vi "LEMP_realtime_v4.vi"() -> ()   [LabVIEW 2019]
uses:
  <vilib>/Analysis/7linalg.llb/Eigenvalue and Vectors Output Option.ctl
  <vilib>/Analysis/baseanly.llb/Matrix Type of Inverse Matrix.ctl
  <vilib>/Analysis/baseanly.llb/Mean (DBL).vi
  <vilib>/Analysis/4window.llb/Hanning Window (DBL).vi
  <vilib>/Analysis/5stat.llb/RMS (DBL).vi
  <vilib>/Analysis/2dsp.llb/Real FFT.vi
  <vilib>/Analysis/7linalg.llb/Real Generalized Eigenvalues and Vectors.vi
  <vilib>/Analysis/7linalg.llb/Real Cholesky Factorization.vi
  <vilib>/Analysis/4window.llb/AllCosWindow (DBL).vi
  <vilib>/Analysis/baseanly.llb/Full Cholesky Factorization.vi
  <vilib>/Analysis/baseanly.llb/Full Real Matrix Cholesky Factorization.vi
  <vilib>/Analysis/Matrix/Numeric/Conversions/Array To Matrix - RA2.vi
  <vilib>/Analysis/baseanly.llb/Real Inverse Matrix.vi
  <vilib>/Analysis/Matrix/Numeric/Multiply/Multiply - RM,RM.vi
  <vilib>/Analysis/7linalg.llb/Real Eigenvalues and Vectors.vi
  <vilib>/Analysis/Matrix/Numeric/Add/Add - RM,RM.vi
  <vilib>/gmath/statdist.llb/Normal Moments.vi
  <vilib>/gmath/NI_Gmath.lvlib
  <vilib>/Analysis/NI_AALPro.lvlib
  <vilib>/Analysis/Matrix/NI_Matrix.lvlib
  <vilib>/Analysis/NI_AALBase.lvlib
panel:
  out "min value":dbl=40.777955555555565
  out "max value":dbl=69.90506666666668
  in  "MASTER":bool
  in  "Tab Control":T1(tab)=enum."Check"
  out "Cycle time (ms)":dbl=0.147275536505731
  out "1st Nat. Freq. (Hz) 2":dbl=40.777955555555565 format="%#_5g"
  out "FEA Frequencies":dbl[](array[numeric])=[47.056894447356875, 51.47067845292848, 50.76081786160022]
  out "Acceleration Data":dbl[](graph) caption="Accelorometer data"
  in  "Real-Time plotting":bool
  out "Probability Density Function":cluster{i32[], dbl[]}(graph)={[9, 10, 11, 12, 13, 14, 15, 16, 17, 18, 19, 20, 21, 22, 23, 24, 25, 26], [0.09171563397251428, 0.12108231855717679, 0.143041857841436, 0.1512135165862316, 0.143041857841436, 0.12108231855717679, 0.09171563397251428, 0.062165735159412254, 0.03770542435775916, 0.020464524096401888, 0.009939041952144324, 0.004319489826678621, 0.0016798304322918924, 0.0005845793791312176, 0.00018203990329545533, 5.072648364839732e-05, 1.2648760741233286e-05, 2.8223200098705454e-06]}
  out "FFT":dbl[](graph)
  out "Frequencies":dynamicdata(graph)=[{"t0"=timestamp(0 s since 1904-01-01), "dt"=1.0, "Y"=array[322 elements]}, {"t0"=timestamp(0 s since 1904-01-01), "dt"=1.0, "Y"=array[322 elements]}]
  out "Position":dynamicdata(graph)=[{"t0"=timestamp(0 s since 1904-01-01), "dt"=1.0, "Y"=[10.0, 12.0, 10.0, 10.0, 10.0, 9.0, 10.0, 12.0, 10.0, 9.0, 9.0, 12.0, 10.0, 16.0, 11.0, 14.0, 14.0, 12.0, 12.0, 12.0, 12.0, 14.0, 14.0, 11.0, 12.0, 12.0, 12.0, 12.0, 12.0, 10.0, 12.0, 14.0, 13.0, 16.0, 14.0, 13.0, 16.0, 14.0, 11.0, 11.0, 16.0, 18.0, 11.0, 10.0, 10.0, 12.0, 10.0, 10.0, 12.0, 12.0, 10.0, 12.0, 10.0, 10.0, 10.0, 10.0, 12.0, 9.0, 11.0, 13.0, 15.0, 15.0, 16.0, 18.0, 15.0, 15.0, 17.0, 15.0, 20.0, 18.0, 15.0, 15.0, 11.0, 11.0, 11.0, 12.0, 9.0, 10.0, 10.0, 10.0, 10.0, 12.0, 14.0, 10.0, 12.0, 12.0, 10.0, 10.0, 10.0, 10.0, 10.0, 10.0, 9.0, 10.0, 12.0, 9.0, 9.0, 14.0, 11.0, 13.0, 15.0, 19.0, 19.0, 17.0, 17.0, 17.0, 21.0, 19.0, 26.0, 26.0, 26.0, 26.0, 24.0, 26.0, 24.0, 24.0, 21.0, 20.0, 20.0, 20.0, 22.0, 14.0, 16.0, 18.0, 18.0, 12.0, 10.0, 12.0, 12.0, 12.0, 16.0, 14.0, 10.0, 14.0, 16.0, 16.0, 20.0, 20.0, 22.0, 22.0, 26.0, 21.0, 19.0, 19.0, 15.0, 19.0, 19.0, 19.0, 19.0, 17.0, 20.0, 24.0, 23.0, 21.0, 21.0, 26.0, 26.0, 26.0, 26.0, 24.0, 24.0, 22.0, 20.0, 22.0, 24.0, 22.0, 24.0, 20.0, 17.0, 18.0, 16.0, 13.0, 14.0, 14.0, 12.0, 10.0, 9.0, 10.0, 11.0, 17.0, 17.0, 24.0, 21.0, 23.0, 24.0, 19.0, 21.0, 25.0, 23.0, 26.0, 25.0, 25.0, 23.0, 23.0, 21.0, 23.0, 25.0, 21.0, 26.0, 24.0, 22.0, 18.0, 14.0, 12.0, 12.0, 12.0, 10.0, 12.0, 10.0, 9.0, 10.0, 10.0, 12.0, 11.0, 10.0, 12.0, 10.0, 10.0, 10.0, 10.0, 10.0, 10.0, 10.0, 9.0, 12.0, 12.0, 11.0, 13.0, 14.0, 12.0, 12.0, 12.0, 10.0, 10.0, 12.0, 10.0, 10.0, 10.0, 9.0, 9.0, 10.0, 12.0, 12.0, 18.0, 14.0, 18.0, 15.0, 12.0, 12.0, 12.0, 14.0, 11.0, 12.0, 12.0, 12.0, 11.0, 10.0, 10.0, 9.0, 10.0, 14.0, 16.0, 12.0, 12.0, 13.0, 13.0, 15.0, 13.0, 14.0, 9.0, 9.0, 10.0, 10.0, 9.0, 10.0, 11.0, 10.0, 10.0, 12.0, 11.0, 14.0, 14.0, 12.0, 12.0, 10.0, 13.0, 15.0, 13.0, 15.0, 15.0, 21.0, 19.0, 16.0, 16.0, 14.0, 16.0, 14.0, 12.0, 10.0, 10.0, 10.0, 10.0, 14.0, 22.0, 24.0, 22.0, 26.0, 22.0, 20.0, 20.0, 19.0, 21.0, 21.0, 17.0, 19.0, 17.0, 16.0, 17.0, 14.0, 12.0, 12.0, 10.0]}, {"t0"=timestamp(0 s since 1904-01-01), "dt"=1.0, "Y"=[9.0, 9.0, 9.0, 10.0, 11.0, 11.0, 12.0, 12.0, 12.0, 12.0, 11.0, 11.0, 10.0, 10.0, 9.0, 9.0, 9.0, 9.0, 10.0, 10.0, 11.0, 11.0, 11.0, 12.0, 12.0, 13.0, 13.0, 14.0, 14.0, 14.0, 14.0, 14.0, 15.0, 15.0, 15.0, 14.0, 13.0, 13.0, 12.0, 11.0, 10.0, 10.0, 10.0, 9.0, 9.0, 9.0, 9.0, 9.0, 10.0, 11.0, 11.0, 12.0, 12.0, 13.0, 14.0, 15.0, 16.0, 16.0, 16.0, 17.0, 17.0, 17.0, 17.0, 17.0, 17.0, 17.0, 16.0, 16.0, 15.0, 15.0, 14.0, 13.0, 12.0, 11.0, 11.0, 10.0, 10.0, 10.0, 9.0, 9.0, 9.0, 9.0, 9.0, 9.0, 9.0, 10.0, 11.0, 12.0, 12.0, 13.0, 14.0, 14.0, 15.0, 15.0, 16.0, 17.0, 18.0, 19.0, 19.0, 19.0, 20.0, 20.0, 20.0, 20.0, 20.0, 19.0, 19.0, 19.0, 18.0, 18.0, 17.0, 16.0, 15.0, 15.0, 14.0, 13.0, 12.0, 11.0, 11.0, 10.0, 10.0, 10.0, 9.0, 9.0, 9.0, 9.0, 9.0, 10.0, 10.0, 11.0, 12.0, 13.0, 14.0, 15.0, 16.0, 18.0, 19.0, 20.0, 21.0, 21.0, 22.0, 22.0, 22.0, 23.0, 23.0, 23.0, 23.0, 23.0, 22.0, 22.0, 22.0, 21.0, 21.0, 20.0, 19.0, 18.0, 16.0, 15.0, 14.0, 13.0, 12.0, 12.0, 12.0, 11.0, 10.0, 10.0, 9.0, 9.0, 9.0, 9.0, 10.0, 10.0, 11.0, 12.0, 13.0, 15.0, 16.0, 18.0, 20.0, 21.0, 22.0, 23.0, 24.0, 25.0, 25.0, 25.0, 25.0, 25.0, 25.0, 25.0, 24.0, 23.0, 22.0, 21.0, 20.0, 19.0, 17.0, 15.0, 14.0, 13.0, 12.0, 11.0, 10.0, 10.0, 9.0, 9.0, 9.0, 9.0, 9.0, 9.0, 9.0, 9.0, 9.0, 9.0, 9.0, 9.0, 9.0, 10.0, 11.0, 11.0, 10.0, 9.0, 9.0, 9.0, 9.0, 9.0, 9.0, 9.0, 9.0, 9.0, 9.0, 9.0, 9.0, 9.0, 9.0, 9.0, 9.0, 9.0, 9.0, 9.0, 10.0, 13.0, 14.0, 13.0, 11.0, 10.0, 9.0, 9.0, 9.0, 9.0, 9.0, 9.0, 9.0, 9.0, 9.0, 9.0, 9.0, 9.0, 9.0, 9.0, 9.0, 10.0, 14.0, 16.0, 17.0, 14.0, 12.0, 10.0, 9.0, 9.0, 9.0, 9.0, 9.0, 9.0, 9.0, 9.0, 9.0, 9.0, 9.0, 9.0, 9.0, 9.0, 10.0, 14.0, 18.0, 19.0, 20.0, 18.0, 14.0, 10.0, 9.0, 9.0, 9.0, 9.0, 9.0, 9.0, 9.0, 9.0, 9.0, 9.0, 9.0, 9.0, 9.0, 9.0, 9.0, 10.0, 13.0, 18.0, 22.0, 22.0, 19.0, 15.0, 12.0, 10.0, 9.0, 9.0, 9.0, 9.0, 9.0, 9.0, 9.0, 9.0]}]
  in  "PDF":bool
  out "Low-Energy Warning":bool
  in  "Frequency Method":enum16{"0-Tone", "1-FFT-CPU", "2-Custom Filter"}(ring)=enum."1-FFT-CPU"
  in  "Width":dbl=0.0508 format="%#.6f"
  in  "Density":dbl=7900.0
  in  "Height":dbl=0.00635
  in  "Length of Beam":dbl=0.3525
  in  "Young's Modulus":dbl=209500000000.0
  in  "Torsion Spring":dbl format="%#.6f"
  in  "Initial Pin node":i32
  in  "Std. Dev.":dbl=0.5 min=0.0
  in  "Eigenvalue Method":T2(ring)
  out "average cycle time (ms)":dbl=4.283940110367686 format="%0.2f"
  in  "FFT data length (data points)":i32=15000
  in  "Min. FFT Power Value (RMS)":dbl=0.02
  in  "Bound to 1st Frequency":bool=TRUE
  in  "accelerometer_mass":dbl=0.055
  in  "Std. Dev = Number of Particles / 3":bool=TRUE
  out "Std. Dev.  2":dbl=1.0
  in  "Number Of Particles":i32=3
  in  "FEA Nodes":i32=60
  in  "file name":i32
  out "FFT_data_length":i32=15000
  in  "Auto FFT length":bool
  out "Hz / per pin location":dbl=1.0
  out "FFT_frequency_resolution":dbl=1.7066666666666668
  in  "scaling_factor_Hz_per_pin_to_frequency_resolution":dbl=0.33 caption="Scale FFT Factor" format="%#_13g"
  in  "Save Acceleration Data":bool=TRUE
  in  "Mode Count":i32=3 min=1 max=10 step=1
  in  "Max Roller Velocity":dbl=3.32
  in  "Buffer seconds":dbl=0.8 min=0.0 max=3.0
  out "acc data":i32=25696
  in  "Frequency selection method":T3(ring)
  in  "Use Top N freq components":i32=5 min=1 max=50 step=1
  in  "Standard Dev":bool=TRUE
  out "Std. Dev. 2":dbl=1.0
  out "1st Nat. Freq. (Hz) 4":waveform(dbl)[](graph)=[{"t0"=timestamp(0 s since 1904-01-01), "dt"=0.004283940110367686, "Y"=array[2994 elements]}, {"t0"=timestamp(0 s since 1904-01-01), "dt"=0.004283940110367686, "Y"=array[2994 elements]}] caption="1st Nat. Freq. (Hz)"
  out "1st Nat. Freq. (Hz) 5":waveform(dbl)[](graph)=[{"t0"=timestamp(0 s since 1904-01-01), "dt"=0.004283940110367686, "Y"=array[2994 elements]}, {"t0"=timestamp(0 s since 1904-01-01), "dt"=0.004283940110367686, "Y"=array[2994 elements]}] caption="1st Nat. Freq. (Hz)"
  # "Note: All Inputs are based on base SI units."
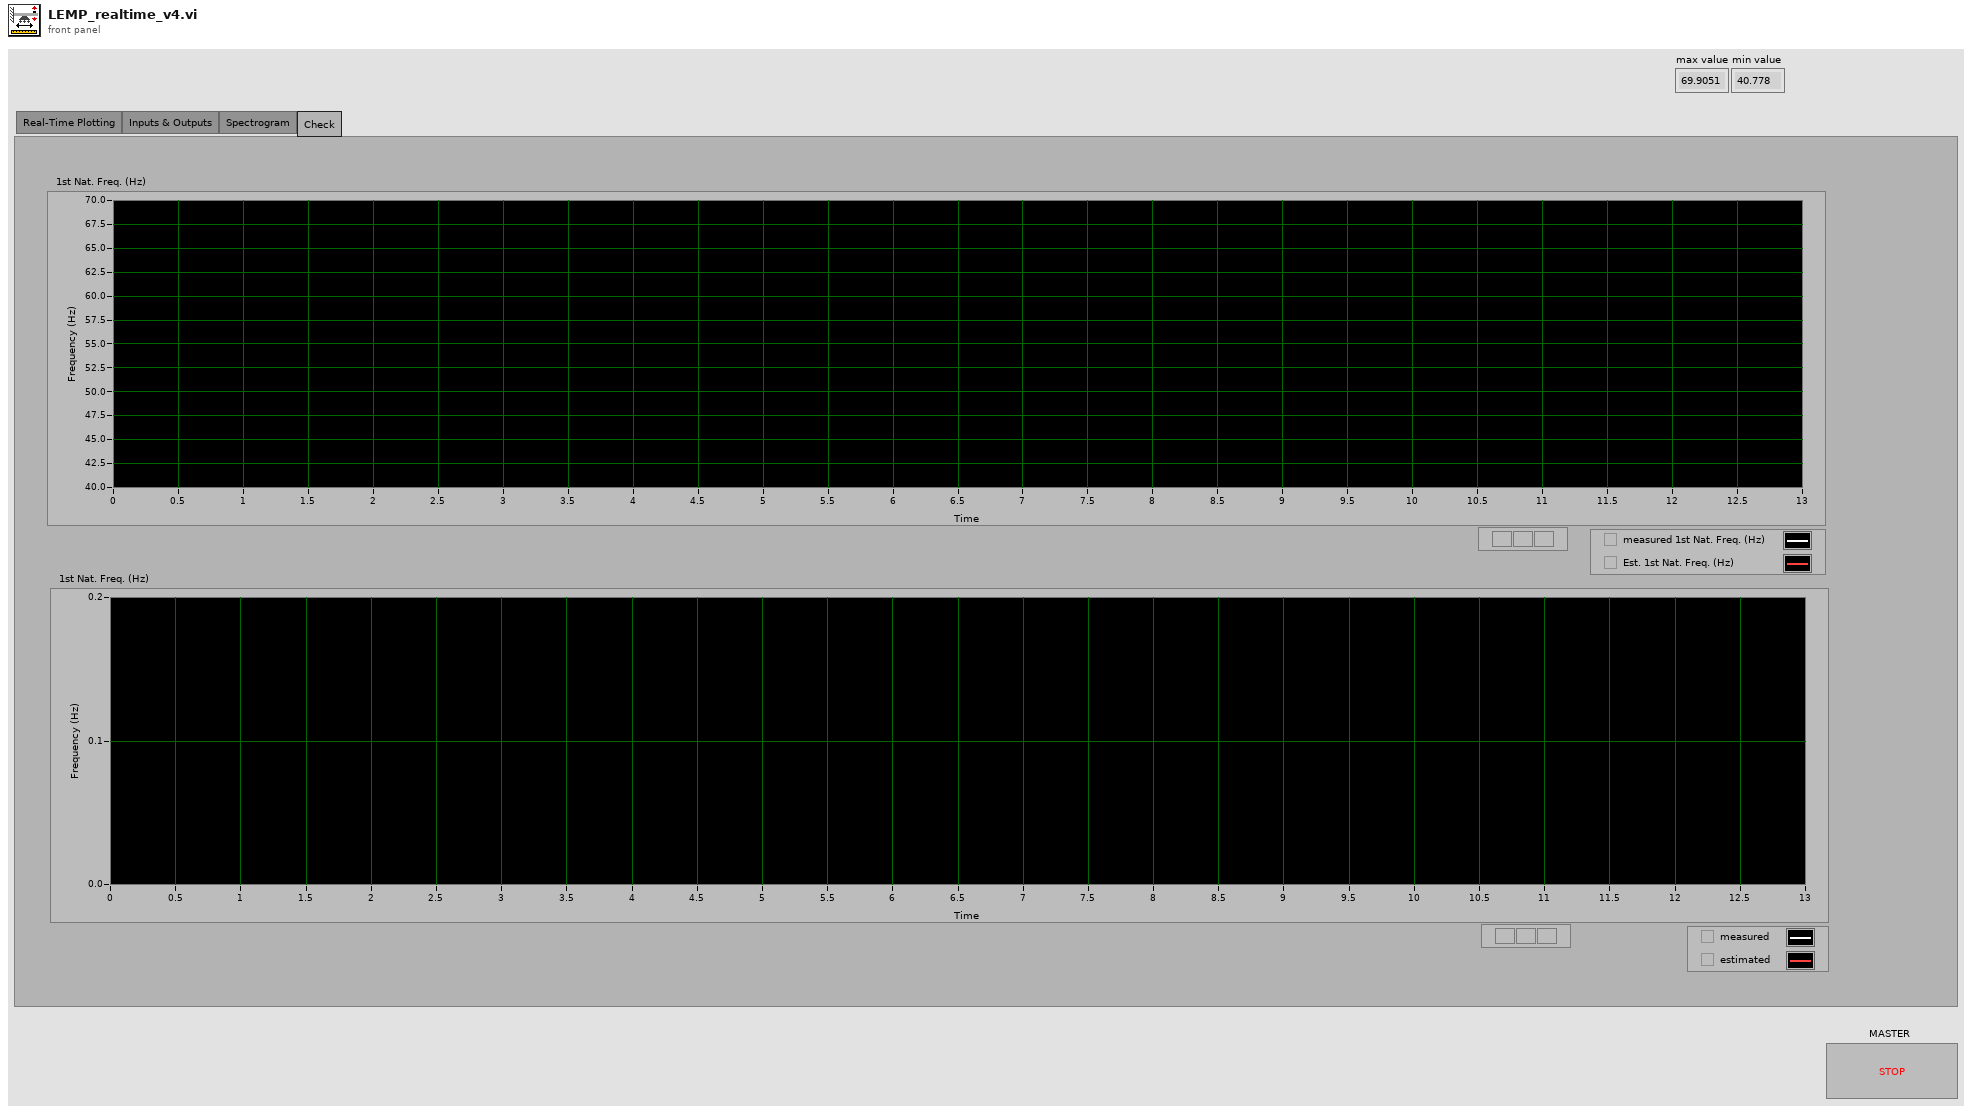
[diagram p1: front panel]
types:
  T1 = enum32{"Real-Time Plotting", "Inputs & Outputs", "Spectrogram", "Check"}
  T2 = enum16{"0-Local Eigen Modification Procedure", "1-LabVIEW generalized eigenvalues", "2-LabVIEW M^-1K eigenvalues", "3-LabVIEW Cholesky Factorization", "4-Cholesky Factorization CPU SGL", "5-Cholesky Factorization CPU FXP", "6-Cholesky Factorization FPGA SGL", "7-Cholesky Factorization FPGA SGL SCL"}
  T3 = enum16{"0-Nearest component to prior ", "1-Coerce maximum differential", "2-Average with nearest component", "3-Top by power", "4-Lowest major component", "5-Average with lowest component"}
  T4 = cluster{"beam_length":dbl, "youngs_modulus":dbl, "torsion_spring":dbl, "beam_height":dbl, "beam_width":dbl, "beam_density":dbl, "number_of_FEA_nodes":i32, "FFT_data_length":i32, "standard_deviation":dbl, "number_of_particles":i32, "min_FFT_power_value":dbl, "initial_pin_node":i32, "accelerometer_mass":dbl, "Max Roller Velocity":dbl}
  T5 = cluster{"beam_length":dbl, "youngs_modulus":dbl, "torsion_spring":dbl, "beam_height":dbl, "beam_width":dbl, "beam_density":dbl, "number_of_FEA_nodes":i32, "FFT_data_length":i32, "standard_deviation":dbl, "number_of_particles":i32, "min_FFT_power_value":dbl, "initial_pin_node":i32, "accelerometer_mass":dbl}
  T6 = cluster{"time_average_cycle":dbl, "measured_frequency":dbl[], "date_time":string, "estimated_pin_node":i32[], "time_cycle_start":dbl[], "measured_pin_location":dbl[], "estimated_frequency":dbl[], "acceleration_data":dbl[], "accelerometer_sample_rate":dbl, "displacement_sample_rate":dbl, "time_compare_start":dbl[], "time_subsample_start":dbl[], "time_FEA_start":dbl[], "time_FEA_end":dbl[], "time_cycle_end":dbl[], "time_accelerometer_aquire_start":dbl[], "time_frequency_calculations_start":dbl[], "time_frequency_calculations_end":dbl[], "measured_pin_location_tt":dbl[], "time_ACC_data_collection_start":dbl, "time_acceleration_data":dbl[], "estimated_pin_location":dbl[], "scaling_factor_Hz_per_pin_to_frequency_resolution":dbl, "Std_Dev_equale_particles_divided_3":bool, "Auto_FFT_length":bool, "windowed_acc_data":dbl[][], "FFT":dbl[][]}
  T7 = cluster{"Eigenvalues":dbl[], "Square Transpose Eigenvectors":dbl[][], "1/deltaStiff":dbl}
  T8 = cluster{"Max frequency":dbl, "Min frequency":dbl, "Max frequency delta per node":dbl, "Max frequency delta per second":dbl}
  T9 = typedef "NI_AALBase.lvlib/Matrix Type of Inverse Matrix.ctl" = enum32{"General", "Positive Definite", "Lower Triangular", "Upper Triangular"}
  T10 = typedef "NI_AALPro.lvlib/Eigenvalue and Vectors Output Option.ctl" = i32
  T11 = typedef "NI_Matrix.lvlib/RealMatrix.ctl" = dbl[][]
  T12 = cluster{"nodes of interest":i32[], "Sample PDF":dbl[]}
  T13 = cluster{"measured_pin_location_tt":dbl[], "measured_pin_location":dbl[]}
  T14 = cluster{"time_acceleration_data":dbl[], "acceleration_data":dbl[]}
  T15 = cluster{"time_cycle_end":dbl[], "estimated_pin_location":dbl[]}
  T16 = cluster{"time_average_cycle":dbl, "measured_frequency":dbl[], "date_time":string, "estimated_pin_node":i32[], "time_cycle_start":dbl[], "measured_pin_location":dbl[], "estimated_frequency":dbl[], "acceleration_data":dbl[], "accelerometer_sample_rate":dbl, "displacement_sample_rate":dbl, "time_compare_start":dbl[], "time_subsample_start":dbl[], "time_FEA_start":dbl[], "time_FEA_end":dbl[], "time_cycle_end":dbl[], "time_accelerometer_aquire_start":dbl[], "time_frequency_calculations_start":dbl[], "time_frequency_calculations_end":dbl[], "measured_pin_location_tt":dbl[], "time_ACC_data_collection_start":dbl, "time_acceleration_data":dbl[], "estimated_pin_location":dbl[], "scaling_factor_Hz_per_pin_to_frequency_resolution":dbl, "Std_Dev_equale_particles_divided_3":bool, "Auto_FFT_length":bool, "windowed_acc_data":dbl[][], "FFT":dbl[][], "beam_length":dbl, "youngs_modulus":dbl, "torsion_spring":dbl, "beam_height":dbl, "beam_width":dbl, "beam_density":dbl, "number_of_FEA_nodes":i32, "FFT_data_length":i32, "standard_deviation":dbl, "number_of_particles":i32, "min_FFT_power_value":dbl, "initial_pin_node":i32, "accelerometer_mass":dbl}
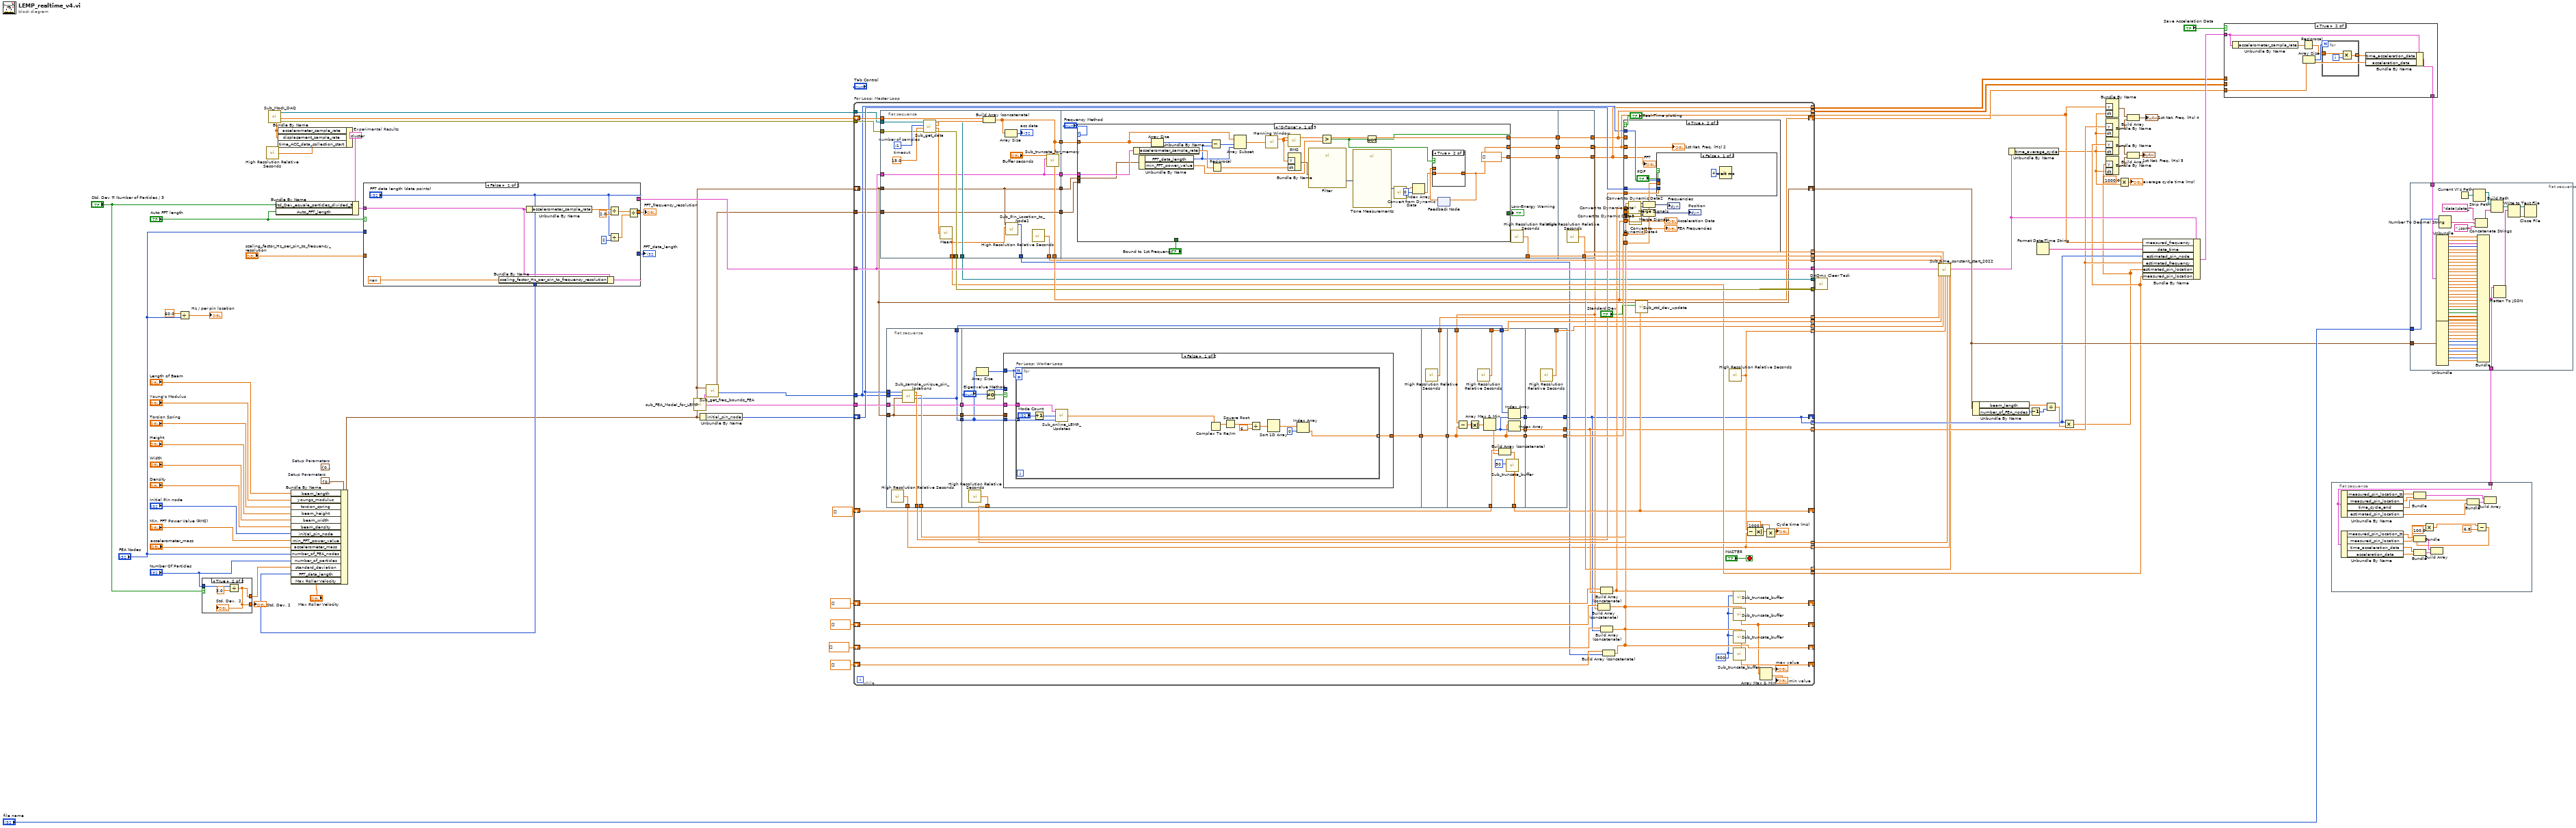
[diagram p0: block diagram]
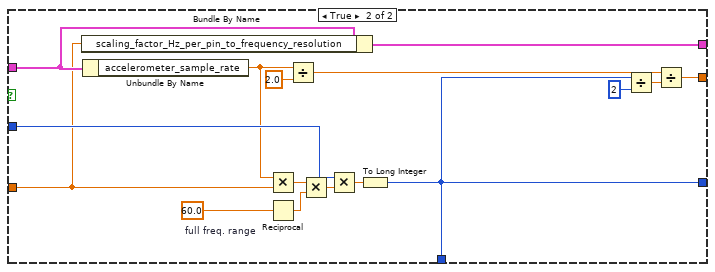
[diagram p3: hidden frame]
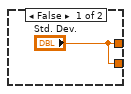
[diagram p4: hidden frame]
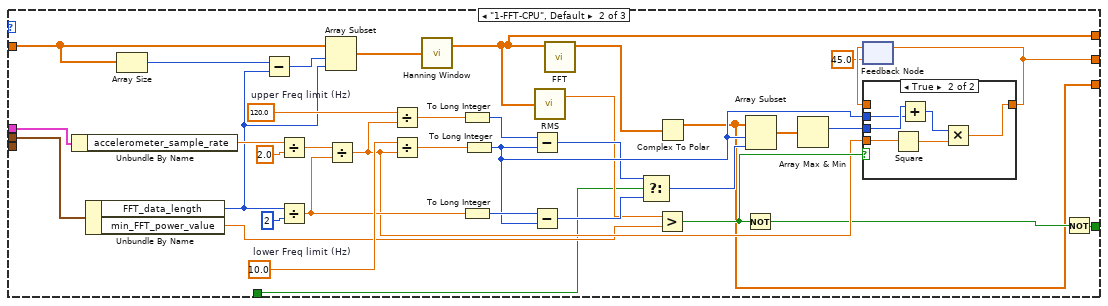
[diagram p6: hidden frame]
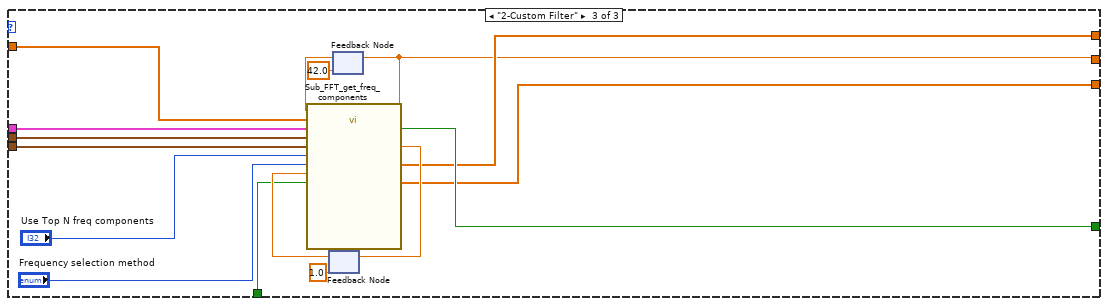
[diagram p8: hidden frame]
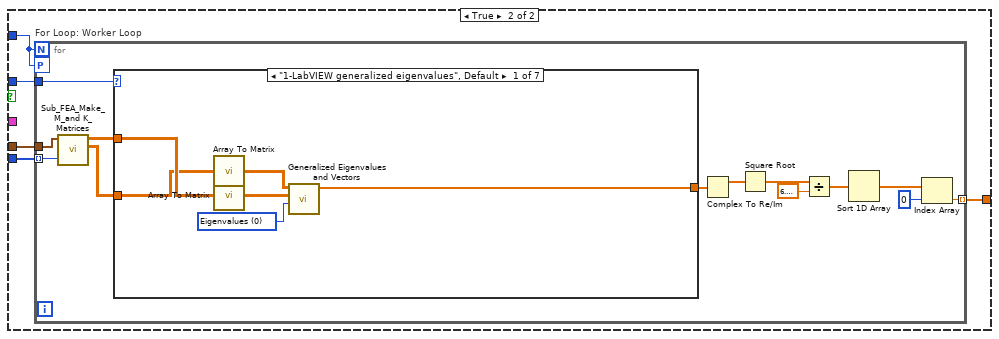
[diagram p9: hidden frame]
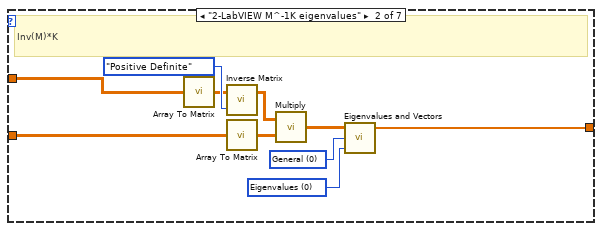
[diagram p10: hidden frame]
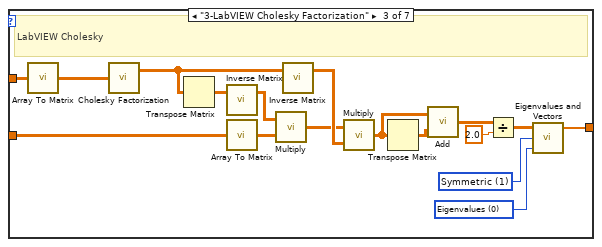
[diagram p11: hidden frame]
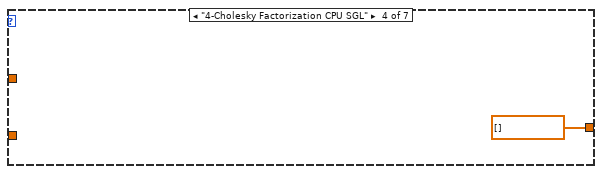
[diagram p12: hidden frame]
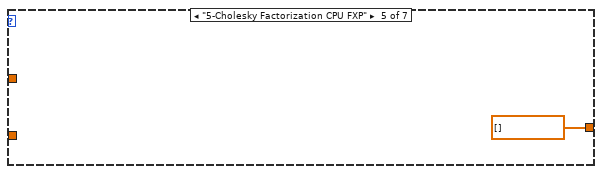
[diagram p13: hidden frame]
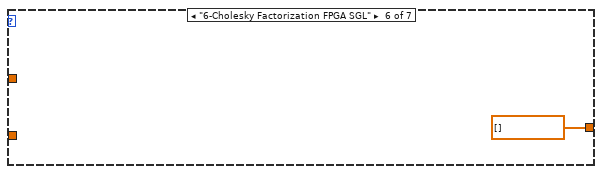
[diagram p14: hidden frame]
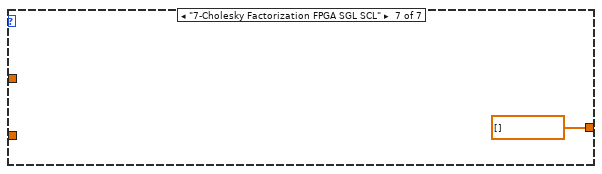
[diagram p15: hidden frame]
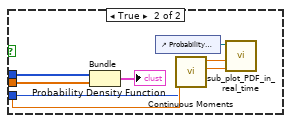
[diagram p17: hidden frame]
diagram:
  w19 = T4 {"beam_length"=0.0, "youngs_modulus"=0.0, "torsion_spring"=0.0, "beam_height"=0.0, "beam_width"=0.0, "beam_density"=0.0, "number_of_FEA_nodes"=0, "FFT_data_length"=0, "standard_deviation"=0.0, "number_of_particles"=0, "min_FFT_power_value"=0.0, "initial_pin_node"=0, "accelerometer_mass"=0.0, "Max Roller Velocity"=0.0}  # Setup Parameters
  (unwired) T5 {"beam_length"=0.0, "youngs_modulus"=0.0, "torsion_spring"=0.0, "beam_height"=0.0, "beam_width"=0.0, "beam_density"=0.0, "number_of_FEA_nodes"=0, "FFT_data_length"=0, "standard_deviation"=0.0, "number_of_particles"=0, "min_FFT_power_value"=0.0, "initial_pin_node"=0, "accelerometer_mass"=0.0}  # Setup Parameters
  w54 = T6 {"time_average_cycle"=0.0, "measured_frequency"=[], "date_time"="", "estimated_pin_node"=[], "time_cycle_start"=[], "measured_pin_location"=[], "estimated_frequency"=[], "acceleration_data"=[], "accelerometer_sample_rate"=0.0, "displacement_sample_rate"=0.0, "time_compare_start"=array[564 elements], "time_subsample_start"=array[564 elements], "time_FEA_start"=array[564 elements], "time_FEA_end"=array[564 elements], "time_cycle_end"=array[564 elements], "time_accelerometer_aquire_start"=array[564 elements], "time_frequency_calculations_start"=array[564 elements], "time_frequency_calculations_end"=array[564 elements], "measured_pin_location_tt"=array[564 elements], "time_ACC_data_collection_start"=0.0, "time_acceleration_data"=array[564 elements], "estimated_pin_location"=array[564 elements], "scaling_factor_Hz_per_pin_to_frequency_resolution"=1.0, "Std_Dev_equale_particles_divided_3"=TRUE, "Auto_FFT_length"=TRUE, "windowed_acc_data"=array1x564[564 elements], "FFT"=array1x564[564 elements]}  # Experimental Results
  n1 = Divide(x=60.0, y="FEA Nodes") -> (x/y=→"Hz / per pin location":dbl)
  n2 = case shown="True" "Std. Dev = Number of Particles / 3" {
    tunnel: ["Std. Dev." w86] -> w34
    tunnel: "Number Of Particles" -> [_ w87]
    tunnel: ["Std. Dev." w86] -> w84
    frame False {
    }
    frame True {
      n3 = Divide(x=w87, y=3.0) -> (x/y=w86:dbl)
      "Std. Dev.  2" <- w86
    }
  }
  "Std. Dev. 2" <- w84
  n4 = call <vilib>:"High Resolution Relative Seconds.vi"() -> ("relative seconds"=w1:dbl)
  n5 = call "Sub_Mock_DAQ.vi"() -> ("DAQ task"=w23:refnum<k21>, "Sample rate"=w20:dbl, "acc data"=w22:dbl[], "error out"=w21:errorcluster)  [unwired: 7 in]
  n6 = Bundle By Name(cluster=w54, "accelerometer_sample_rate"=w20, "displacement_sample_rate"=w20, "time_ACC_data_collection_start"=w1) -> (w48:T6)
  n7 = Bundle By Name(cluster=w48, "Std_Dev_equale_particles_divided_3"="Std. Dev = Number of Particles / 3", "Auto_FFT_length"="Auto FFT length") -> (w45:T6)
  n8 = case shown="False" "Auto FFT length" {
    tunnel: "FEA Nodes" -> [_ w106]
    tunnel: w45 -> [w92 w103]
    tunnel: ["FFT data length (data points)" w101] -> w35
    tunnel: [w93 w105] -> w53
    tunnel: ["FFT data length (data points)" w101] -> w52
    tunnel: [w91 w102] -> w49
    tunnel: "scaling_factor_Hz_per_pin_to_frequency_resolution" -> [_ w100]
    frame False {
      n9 = Bundle By Name(cluster=w92, "scaling_factor_Hz_per_pin_to_frequency_resolution"=nan) -> (w91:T6)
      n10 = Unbundle By Name(w92) -> ("accelerometer_sample_rate"=w98:dbl)
      n11 = Divide(x=w98, y=2.0) -> (x/y=w96:dbl)
      n12 = Divide(x="FFT data length (data points)", y=2) -> (x/y=w97:dbl)
      n13 = Divide(x=w96, y=w97) -> (x/y=w93:dbl)
    }
    frame True {
      w109 = 60.0  # full freq. range
      n14 = Bundle By Name(cluster=w103, "scaling_factor_Hz_per_pin_to_frequency_resolution"=w100) -> (w102:T6)
      n15 = Unbundle By Name(w103) -> ("accelerometer_sample_rate"=w99:dbl)
      n16 = Multiply(x=w99, y=w100) -> (x*y=w112:dbl)
      n17 = Reciprocal(x=w109) -> (1/x=w113:dbl)
      n18 = Divide(x=w99, y=2.0) -> (x/y=w110:dbl)
      n19 = Multiply(x=w112, y=w113) -> (x*y=w114:dbl)
      n20 = Multiply(x=w106, y=w114) -> (x*y=w104:dbl)
      n21 = To Long Integer(number=w104) -> (32bit integer=w101:i32)
      n22 = Divide(x=w101, y=2) -> (x/y=w111:dbl)
      n23 = Divide(x=w110, y=w111) -> (x/y=w105:dbl)
    }
  }
  "FFT_frequency_resolution" <- w53
  "FFT_data_length" <- w52
  n24 = Bundle By Name(cluster=w19, "beam_length"="Length of Beam", "youngs_modulus"="Young's Modulus", "torsion_spring"="Torsion Spring", "beam_height"="Height", "beam_width"="Width", "beam_density"="Density", "initial_pin_node"="Initial Pin node", "min_FFT_power_value"="Min. FFT Power Value (RMS)", "accelerometer_mass"="accelerometer_mass", "number_of_FEA_nodes"="FEA Nodes", "number_of_particles"="Number Of Particles", "standard_deviation"=w34, "FFT_data_length"=w35, "Max Roller Velocity"="Max Roller Velocity") -> (w15:T4)
  n25 = call "sub_FEA_Model_for_LEMP.vi"("Setup Parameters"=w15) -> ("LEMP"=w14:T7)
  n26 = Unbundle By Name(w15) -> ("initial_pin_node"=w73:i32)
  n27 = call "Sub_get_freq_bounds_FEA.vi"("Setup Parameters"=w15, "LEMP"=w14) -> ("Beam frequency params"=w16:T8, "nodes of interest"=w13:i32[])  [unwired: 2 out]
  n28 = while "For Loop: Master Loop" {
    shift-right: [w126] -> _
    shift-left: w73 -> [w180]
    tunnel: [w139] -> w27 mode=indexing
    tunnel: w13 -> [w143]
    tunnel: [w126] -> w28 mode=indexing
    tunnel: w23 -> [w173]
    tunnel: [w170] -> w82
    tunnel: [w171] -> w81
    shift-right: [w174] -> w41
    shift-left: w22 -> [w175]
    tunnel: [w137] -> w5 mode=indexing
    tunnel: w49 -> [w184]
    tunnel: [w184] -> w61
    tunnel: w21 -> [w172]
    tunnel: [w124] -> w66 mode=indexing
    tunnel: [w164] -> w29 mode=indexing
    tunnel: [w163] -> w69 mode=indexing
    tunnel: [w153] -> w64 mode=indexing
    tunnel: [w162] -> w67 mode=indexing
    tunnel: [w161] -> w68 mode=indexing
    tunnel: [w122] -> w70 mode=indexing
    tunnel: [w158] -> w63 mode=indexing
    tunnel: [w125] -> w65 mode=indexing
    tunnel: [w156] -> w26 mode=indexing
    tunnel: [w142] -> w25 mode=indexing
    tunnel: w14 -> [w154]
    tunnel: [w152] -> w4 mode=indexing
    tunnel: [w153] -> w24 mode=indexing
    tunnel: w16 -> [w151]
    shift-right: [w144] -> _
    shift-left: dbl[] [] ("array") -> [w147]
    shift-right: [w145] -> w59
    shift-left: w15 -> [w146]
    shift-right: [w140] -> _
    shift-left: dbl[] [] ("array") -> [w141]
    shift-right: [w115] -> _
    shift-left: dbl[] [] ("array") -> [w138]
    shift-right: [w134] -> _
    shift-left: dbl[] [] ("array") -> [w132]
    shift-right: [w116] -> _
    shift-left: dbl[] [] ("array") -> [w133]
    stop <- "MASTER" stop-if-true
    w128 = 800 ("samples")
    n29 = flat-sequence {
      tunnel: w146 -> [w188]
      tunnel: w184 -> [w192]
      tunnel: [w192] -> w178
      tunnel: [w190] -> w177
      tunnel: [w188] -> w176
      tunnel: w175 -> [w205]
      tunnel: [w193] -> w174
      tunnel: w173 -> [w203]
      tunnel: w172 -> [w201]
      tunnel: [w199] -> w171
      tunnel: [w198] -> w170
      tunnel: [w204] -> w153
      tunnel: [w195] -> w152
      tunnel: w151 -> [w194]
      tunnel: [w194] -> w150
      tunnel: [w187] -> w131
      tunnel: w178 -> [w214]
      tunnel: w177 -> [w213]
      tunnel: w176 -> [w212]
      tunnel: [w216] -> w166
      tunnel: [w211] -> w165
      tunnel: [w209] -> w162
      tunnel: w150 -> [w206]
      tunnel: [w207] -> w148
      tunnel: [w302] -> w137
      tunnel: [w305] -> w156
      tunnel: w166 -> [w305]
      tunnel: w165 -> [w302]
      tunnel: [w304] -> w161
      tunnel: w148 -> [w303]
      tunnel: [w303] -> w142
      frame #0 {
        w196 = 15.0  # timeout
        w202 = -1  # number of samples
        n30 = call "Sub_get_data.vi"("error in"=w201, "timeout"=w196, "number of samples per channel"=w202, "task/channels in"=w203) -> ("error out"=w199:errorcluster, "Pin location meters"=w197:dbl[], "ACC m/s2"=w200:dbl[], "task/channels out"=w198:refnum<k21>)  [unwired: 1 in, 3 out]
        n31 = call-poly <vilib>:"Mean.vi"("X"=w197) -> ("mean"=w195:dbl)  [unwired: 1 out]
        n32 = Build Array (concatenate)(w205, w200) -> (w190:dbl[])
        n33 = Array Size(array=w190) -> (size(s)=→"acc data":i32)
        n34 = call "Sub_Pin_Location_to_Node2.vi"("Pin Location"=w195, "Setup Parameters"=w188) -> ("DOF of Interest"=w187:i32)  [unwired: 9 in]
        n35 = call <vilib>:"High Resolution Relative Seconds.vi"() -> ("relative seconds"=w204:dbl)
        n36 = call "Sub_truncate_for_memory.vi"("ACC m/s2"=w190, "Experimental Results"=w192, "Buffer seconds"="Buffer seconds") -> ("ACC m/s2"=w193:dbl[])  [unwired: 8 in]
      }
      frame #1 {
        n37 = case shown="\"0-Tone\"" "Frequency Method" {
          tunnel: [w227 w245 w288] -> w211
          tunnel: [w229 w244 w291] -> w216
          tunnel: w213 -> [w231 w250 w294]
          tunnel: [w224 w278 w292] -> w215
          tunnel: w212 -> [w220 w249 w296]
          tunnel: w214 -> [w222 w248 w295]
          tunnel: w206 -> [_ _ w297]
          tunnel: "Bound to 1st Frequency" -> [_ w247 w298]
          tunnel: [dbl[] [] ("Real freq comp (out)") w243 w286] -> w207
          frame "0-Tone" {
            n38 = Unbundle By Name(w222) -> ("accelerometer_sample_rate"=w221:dbl)
            n39 = Unbundle By Name(w220) -> ("FFT_data_length"=w218:i32, "min_FFT_power_value"=w219:dbl)
            n40 = Array Size(array=w231) -> (size(s)=w239:i32)
            n41 = Subtract(x=w239, y=w218) -> (x-y=w238:i32)
            n42 = Reciprocal(x=w221) -> (1/x=w223:dbl)
            n43 = Array Subset(array=w231, index=w238, length=w218) -> (w232:dbl[])
            n44 = call-poly <vilib>:"Hanning Window.vi"("X"=w232) -> ("Windowed X"=w229:dbl[])  [unwired: 1 out]
            n45 = Bundle By Name("Y"=w229, "dt"=w223) -> (w233:waveform(dbl))  [unwired: 1 in]
            n46 = call-poly <vilib>:"RMS.vi"("X"=w229) -> ("rms value"=w225:dbl)  [unwired: 1 out]
            n47 = call "Filter"("Signal"=w233) -> ("Filtered Signal"=w234:dynamicdata)  [unwired: 9 in, 1 out]
            n48 = Greater?(x=w225, y=w219) -> (0:w226:bool)
            n49 = call "Tone Measurements"("Signals"=w234) -> ("Frequency"=w235:dynamicdata)  [unwired: 9 in, 1 out]
            n50 = Not(x=w226) -> (.not. x?=w224:bool)
            n51 = call "Convert from Dynamic Data"("Dynamic Data Type"=w235) -> ("Array"=w236:dbl[])  [unwired: 3 in]
            n52 = Index Array(array=w236, index=0) -> (element=w228:dbl)
            n53 = feedback #1() -> (w230:dbl)  [unwired: 1 in]
            n54 = case shown="True" w226 {
              tunnel: [w240 w241] -> w227
              tunnel: w230 -> [w240 _]
              tunnel: w228 -> [_ w241]
              frame False {
              }
              frame True {
              }
            }
            n55 = feedback-in #1(w227) -> ()
          }
          frame "1-FFT-CPU", Default {
            w262 = 120.0  # upper Freq limit (Hz)
            w276 = 10.0  # lower Freq limit (Hz)
            n56 = Unbundle By Name(w248) -> ("accelerometer_sample_rate"=w252:dbl)
            n57 = Unbundle By Name(w249) -> ("FFT_data_length"=w251:i32, "min_FFT_power_value"=w253:dbl)
            n58 = Array Size(array=w250) -> (size(s)=w268:i32)
            n59 = Subtract(x=w268, y=w251) -> (x-y=w267:i32)
            n60 = Divide(x=w252, y=2.0) -> (x/y=w270:dbl)
            n61 = Divide(x=w251, y=2) -> (x/y=w269:dbl)
            n62 = Array Subset(array=w250, index=w267, length=w251) -> (w266:dbl[])
            n63 = Divide(x=w270, y=w269) -> (x/y=w261:dbl)
            n64 = Divide(x=w262, y=w261) -> (x/y=w260:dbl)
            n65 = Divide(x=w276, y=w261) -> (x/y=w275:dbl)
            n66 = call-poly <vilib>:"Hanning Window.vi"("X"=w266) -> ("Windowed X"=w244:dbl[])  [unwired: 1 out]
            n67 = To Long Integer(number=w260) -> (32bit integer=w259:i32)
            n68 = To Long Integer(number=w269) -> (32bit integer=w272:i32)
            n69 = To Long Integer(number=w275) -> (32bit integer=w258:i32)
            n70 = Subtract(x=w259, y=w258) -> (x-y=w256:i32)
            n71 = Subtract(x=w272, y=w258) -> (x-y=w255:i32)
            n72 = call-poly <vilib>:"RMS.vi"("X"=w244) -> ("rms value"=w254:dbl)  [unwired: 1 out]
            n73 = call-poly <vilib>:"FFT.vi"("X"=w244) -> ("FFT {X}"=w273:cdb[])  [unwired: 9 in, 1 out]
            n74 = Select(t=w256, s=w247, f=w255) -> (s? t:f=w257:i32)
            n75 = Greater?(x=w254, y=w253) -> (0:w263:bool)
            n76 = Complex To Polar(r * e^(i*theta)=w273) -> (r=w243:dbl[])  [unwired: 1 out]
            n77 = Not(x=w263) -> (.not. x?=w246:bool)
            n78 = Array Subset(array=w243, index=w258, length=w257) -> (w264:dbl[])
            n79 = Array Max & Min(array=w264) -> (max index (indices)=w274:i32)  [unwired: 3 out]
            n80 = feedback #2(45.0) -> (w265:dbl)
            n81 = case shown="True" w263 {
              tunnel: w274 -> [_ w285]
              tunnel: w258 -> [_ w283]
              tunnel: w261 -> [_ w282]
              tunnel: [w279 w280] -> w245
              tunnel: w265 -> [w279 _]
              frame False {
              }
              frame True {
                n82 = Square(x=w282) -> (x^2=w281:dbl)
                n83 = Add(x=w285, y=w283) -> (x+y=w284:i32)
                n84 = Multiply(x=w284, y=w281) -> (x*y=w280:dbl)
              }
            }
            n85 = feedback-in #2(w245) -> ()
            n86 = Not(x=w246) -> (.not. x?=w278:bool)
          }
          frame "2-Custom Filter" {
            n87 = feedback #3(1.0 ("Slop factor (Feed back)")) -> (w300:dbl)
            n88 = feedback #4(42.0) -> (w299:dbl)
            n89 = call "Sub_FFT_get_freq_components.vi"("Prior Frequency Estimate (Feed forward)"=w299, "ACC Signal"=w294, "Experimental Results"=w295, "Setup Parameters"=w296, "Beam frequency params"=w297, "Use Top N freq components"="Use Top N freq components", "Frequency selection method"="Frequency selection method", "Slop factor (Feed forward)"=w300, "Bound to 1st Frequency"=w298) -> ("Windowed X (out)"=w291:dbl[], "Real freq comp (out)"=w286:dbl[], "Next Frequency Estimate"=w288:dbl, "Low Energy"=w292:bool, "Slop factor (Feed back)"=w301:dbl)  [unwired: 14 in]
            n90 = feedback-in #3(w301) -> ()
            n91 = feedback-in #4(w288) -> ()
          }
        }
        "Low-Energy Warning" <- w215
        n92 = call <vilib>:"High Resolution Relative Seconds.vi"() -> ("relative seconds"=w209:dbl)
      }
      frame #2 {
        n93 = call <vilib>:"High Resolution Relative Seconds.vi"() -> ("relative seconds"=w304:dbl)
      }
    }
    n94 = flat-sequence {
      tunnel: w146 -> [w309]
      tunnel: [w309] -> w183
      tunnel: [w313] -> w182
      tunnel: [w312] -> w181
      tunnel: w180 -> [w311]
      tunnel: [w307] -> w179
      tunnel: [w310] -> w124
      tunnel: w154 -> [w308]
      tunnel: [w308] -> w155
      tunnel: [w307] -> w149
      tunnel: w143 -> [w306]
      tunnel: w183 -> [w320]
      tunnel: [w321] -> w160
      tunnel: [w319] -> w164
      tunnel: w155 -> [w316]
      tunnel: w149 -> [w314]
      tunnel: w160 -> [w394]
      tunnel: [w394] -> w159
      tunnel: [w393] -> w158
      tunnel: w159 -> [w405]
      tunnel: w179 -> [w406]
      tunnel: w137 -> [w404]
      tunnel: [w405] -> w169
      tunnel: [w403] -> w168
      tunnel: [w402] -> w167
      tunnel: [w401] -> w163
      tunnel: [w398] -> w144
      tunnel: w147 -> [w397]
      tunnel: [w410] -> w139
      tunnel: [w411] -> w126
      tunnel: [w412] -> w185
      tunnel: w169 -> [w412]
      tunnel: w168 -> [w411]
      tunnel: w167 -> [w410]
      tunnel: [w409] -> w125
      frame #0 {
        n95 = call <vilib>:"High Resolution Relative Seconds.vi"() -> ("relative seconds"=w310:dbl)
        n96 = call "Sub_sample_unique_pin_locations.vi"("Setup Parameters"=w309, "FEA Nodes"=w306, "Initial Pin Location"=w311) -> ("Unique Samples"=w307:i32[], "Sample PDF"=w313:dbl[], "Standard Deviation"=w312:dbl)  [unwired: 6 in]
      }
      frame #1 {
        n97 = call <vilib>:"High Resolution Relative Seconds.vi"() -> ("relative seconds"=w319:dbl)
        n98 = Array Size(array=w314) -> (size(s)=w315:i32)
        n99 = Not Equal To 0?(x="Eigenvalue Method") -> (x != 0?=w318:bool)
        n100 = case shown="False" w318 {
          tunnel: w314 -> [w324 w342]
          tunnel: [w323 w341] -> w321
          tunnel: w320 -> [_ w340]
          tunnel: w315 -> [w325 w339]
          tunnel: "Eigenvalue Method" -> [_ w338]
          tunnel: w316 -> [w322 _]
          frame False {
            n101 = for "For Loop: Worker Loop" {
              N: w325 -> [_]
              workers-P: w325 -> [_]
              tunnel: w324 -> [w326] mode=indexing
              tunnel: [w331] -> w323 mode=indexing
              tunnel: w322 -> [w329]
              n102 = Increment(x="Mode Count") -> (x+1=w327:i32)
              n103 = call "Sub_online_LEMP_Updatec.vi"("Effected DOF"=w326, "Mode count"=w327, "LEMP"=w329) -> ("Updated Eigenvalues"=w330:dbl[])
              n104 = Complex To Re/Im ("Complex To Cartesian.vi")(x + iy=w330) -> (x=w337:dbl[])  [unwired: 1 out]
              n105 = Square Root ("Square Root.vi")(x=w337) -> (sqrt(x)=w336:dbl[])
              n106 = Divide(x=w336, y=6.283185307179586) -> (x/y=w332:dbl[])
              n107 = Sort 1D Array(array=w332) -> (sorted array=w334:dbl[])
              n108 = Index Array(array=w334, index=0) -> (element=w331:dbl)
            }
          }
          frame True {
            n109 = for "For Loop: Worker Loop" {
              N: w339 -> [_]
              tunnel: [w350] -> w341 mode=indexing
              tunnel: w342 -> [w347] mode=indexing
              tunnel: w340 -> [w343]
              workers-P: w339 -> [_]
              tunnel: w338 -> [w344]
              n110 = call "Sub_FEA_Make_M_and K_Matrices.vi"("Pin Location"=w347, "Setup Parameters"=w343) -> ("K Matrix"=w346:dbl[][], "M Matrix"=w345:dbl[][])  [unwired: 8 in]
              n111 = case shown="\"1-LabVIEW generalized eigenvalues\", Default" w344 {
                tunnel: w345 -> [w359 w365 w373 _ _ _ _]
                tunnel: w346 -> [w358 w363 w375 _ _ _ _]
                tunnel: [w360 w368 w376 cdb[] [] ("Eigenvalues") cdb[] [] ("Eigenvalues") cdb[] [] ("Eigenvalues") cdb[] [] ("Eigenvalues")] -> w348
                frame "1-LabVIEW generalized eigenvalues", Default {
                  w361 = T10 0 items=["Eigenvalues", "Eigenvalues & Vectors"] ("output option")
                  n112 = call-poly <vilib>:"Array To Matrix.vi"("Real 2D Array"=w358) -> ("Real Matrix"=w357:T11)
                  n113 = call-poly <vilib>:"Array To Matrix.vi"("Real 2D Array"=w359) -> ("Real Matrix"=w356:T11)
                  n114 = call-poly <vilib>:"Generalized Eigenvalues and Vectors.vi"("output option"=w361, "B"=w356, "A"=w357) -> ("Eigenvalues"=w360:cdb[])  [unwired: 3 in, 2 out]
                }
                frame "2-LabVIEW M^-1K eigenvalues" {
                  w367 = T10 0 items=["Eigenvalues", "Eigenvalues & Vectors"] ("output option")
                  w370 = 0 items=["General", "Symmetric"] ("matrix type")
                  # "Inv(M)*K"
                  n115 = call-poly <vilib>:"Array To Matrix.vi"("Real 2D Array"=w365) -> ("Real Matrix"=w364:T11)
                  n116 = call-poly <vilib>:"Inverse Matrix.vi"("matrix type"=Matrix_Type_of_Inverse_Matrix."Positive Definite", "Input Matrix"=w364) -> ("Inverse Matrix"=w371:T11)  [unwired: 1 out]
                  n117 = call-poly <vilib>:"Array To Matrix.vi"("Real 2D Array"=w363) -> ("Real Matrix"=w362:T11)
                  n118 = call-poly <vilib>:"Multiply.vi"("Real Matrix B"=w362, "Real Matrix A"=w371) -> ("A * B"=w369:T11)
                  n119 = call-poly <vilib>:"Eigenvalues and Vectors.vi"("output option"=w367, "matrix type"=w370, "Input Matrix"=w369) -> ("Eigenvalues"=w368:cdb[])  [unwired: 2 out]
                }
                frame "3-LabVIEW Cholesky Factorization" {
                  w378 = T10 0 items=["Eigenvalues", "Eigenvalues & Vectors"] ("output option")
                  w379 = 1 items=["General", "Symmetric"] ("matrix type")
                  # "LabVIEW Cholesky"
                  n120 = call-poly <vilib>:"Array To Matrix.vi"("Real 2D Array"=w373) -> ("Real Matrix"=w372:T11)
                  n121 = call-poly <vilib>:"Cholesky Factorization.vi"("A"=w372) -> ("Cholesky"=w387:T11)  [unwired: 1 out]
                  n122 = Transpose Matrix(1:w387) -> (0:w388:T11)
                  n123 = call-poly <vilib>:"Inverse Matrix.vi"("Input Matrix"=w388) -> ("Inverse Matrix"=w386:T11)  [unwired: 1 in, 1 out]
                  n124 = call-poly <vilib>:"Array To Matrix.vi"("Real 2D Array"=w375) -> ("Real Matrix"=w374:T11)
                  n125 = call-poly <vilib>:"Multiply.vi"("Real Matrix B"=w374, "Real Matrix A"=w386) -> ("A * B"=w384:T11)
                  n126 = call-poly <vilib>:"Inverse Matrix.vi"("Input Matrix"=w387) -> ("Inverse Matrix"=w385:T11)  [unwired: 1 in, 1 out]
                  n127 = call-poly <vilib>:"Multiply.vi"("Real Matrix B"=w385, "Real Matrix A"=w384) -> ("A * B"=w383:T11)
                  n128 = Transpose Matrix(1:w383) -> (0:w382:T11)
                  n129 = call-poly <vilib>:"Add.vi"("Real Matrix B"=w382, "Real Matrix A"=w383) -> ("A + B"=w380:T11)
                  n130 = Divide(x=w380, y=2.0) -> (x/y=w377:T11)
                  n131 = call-poly <vilib>:"Eigenvalues and Vectors.vi"("output option"=w378, "matrix type"=w379, "Input Matrix"=w377) -> ("Eigenvalues"=w376:cdb[])  [unwired: 2 out]
                }
                frame "4-Cholesky Factorization CPU SGL" {
                }
                frame "5-Cholesky Factorization CPU FXP" {
                }
                frame "6-Cholesky Factorization FPGA SGL" {
                }
                frame "7-Cholesky Factorization FPGA SGL SCL" {
                }
              }
              n132 = Complex To Re/Im ("Complex To Cartesian.vi")(x + iy=w348) -> (x=w355:dbl[])  [unwired: 1 out]
              n133 = Square Root ("Square Root.vi")(x=w355) -> (sqrt(x)=w354:dbl[])
              n134 = Divide(x=w354, y=6.283185307179586) -> (x/y=w349:dbl[])
              n135 = Sort 1D Array(array=w349) -> (sorted array=w352:dbl[])
              n136 = Index Array(array=w352, index=0) -> (element=w350:dbl)
            }
          }
        }
      }
      frame #2 {
        n137 = call <vilib>:"High Resolution Relative Seconds.vi"() -> ("relative seconds"=w393:dbl)
      }
      frame #3 {
        n138 = Subtract(x=w404, y=w405) -> (x-y=w408:dbl[])
        n139 = Absolute Value(x=w408) -> (abs(x)=w400:dbl[])
        n140 = call <vilib>:"High Resolution Relative Seconds.vi"() -> ("relative seconds"=w401:dbl)
        n141 = Array Max & Min(array=w400) -> (min value=w396:dbl, min index (indices)=w407:i32)  [unwired: 2 out]
        n142 = Build Array (concatenate)(w397, w396) -> (w399:dbl[])
        n143 = call "Sub_truncate_buffer.vi"("array"=w399, "samples"=50) -> ("array"=w398:dbl[])  [unwired: 9 in]
        n144 = Index Array(array=w406, index=w407) -> (element=w403:i32)
        n145 = Index Array(array=w405, index=w407) -> (element=w402:dbl)
      }
      frame #4 {
        n146 = call <vilib>:"High Resolution Relative Seconds.vi"() -> ("relative seconds"=w409:dbl)
      }
    }
    n147 = Build Array (concatenate)(w138, w137) -> (w135:dbl[])
    n148 = Build Array (concatenate)(w141, w139) -> (w136:dbl[])
    n149 = Build Array (concatenate)(w132, w126) -> (w130:dbl[])
    n150 = Build Array (concatenate)(w133, w131) -> (w129:dbl[])
    n151 = case shown="True" "Real-Time plotting" {
      tunnel: w181 -> [_ w431]
      tunnel: w180 -> [_ w430]
      tunnel: w143 -> [_ w429]
      tunnel: w182 -> [_ w428]
      tunnel: w185 -> [_ w427]
      tunnel: w156 -> [_ _]
      tunnel: w174 -> [_ w426]
      tunnel: w137 -> [_ w424]
      tunnel: w142 -> [_ w425]
      tunnel: w136 -> [_ w422]
      tunnel: w135 -> [_ w420]
      tunnel: w130 -> [_ w417]
      tunnel: w129 -> [_ w415]
      frame False {
      }
      frame True {
        n152 = call "Convert to Dynamic Data"("Array"=w422) -> ("Dynamic Data Type"=w421:dynamicdata)  [unwired: 3 in]
        n153 = call "Convert to Dynamic Data2"("Array"=w420) -> ("Dynamic Data Type"=w419:dynamicdata)  [unwired: 3 in]
        n154 = call "Convert to Dynamic Data3"("Array"=w417) -> ("Dynamic Data Type"=w416:dynamicdata)  [unwired: 3 in]
        n155 = call "Convert to Dynamic Data4"("Array"=w415) -> ("Dynamic Data Type"=w414:dynamicdata)  [unwired: 3 in]
        n156 = Merge Signals(w421, w419) -> (→"Frequencies":dynamicdata)
        n157 = Merge Signals(w416, w414) -> (→"Position":dynamicdata)
        n158 = case shown="False" "PDF" {
          tunnel: w431 -> [_ w440]
          tunnel: w430 -> [_ w439]
          tunnel: w429 -> [_ w438]
          tunnel: w428 -> [_ w437]
          frame False {
            n159 = Wait (ms)(milliseconds to wait=u32 4) -> ()  [unwired: 1 out]
          }
          frame True {
            n160 = Bundle("nodes of interest"=w438, "Sample PDF"=w437) -> (→"Probability Density Function":T12)  [unwired: 1 in]
            n161 = control-ref of="Probability Density Function"() -> (w434:refnum<vi>)
            n162 = call-poly <vilib>:"Continuous Moments.vi"("std"=w440, "mean"=w439) -> ("variance"=w435:dbl, "mean"=w433:dbl)  [unwired: 7 in, 1 out]
            n163 = call "sub_plot_PDF_in_real_time.vi"("mean"=w433, "variance"=w435, "XYGraph in"=w434) -> ()  [unwired: 9 in]
          }
        }
        "FEA Frequencies" <- w427
        "Acceleration Data" <- w426
        "1st Nat. Freq. (Hz) 2" <- w424
        "FFT" <- w425
      }
    }
    n164 = call "Sub_std_dev_update.vi"("Frequency differentials"=w144, "standard dev"="Standard Dev", "Setup Parameters"=w146) -> ("Setup Parameters"=w145:T4)  [unwired: 8 in]
    n165 = call <vilib>:"High Resolution Relative Seconds.vi"() -> ("relative seconds"=w122:dbl)
    n166 = call "Sub_truncate_buffer.vi"("array"=w136, "samples"=w128) -> ("array"=w140:dbl[])  [unwired: 9 in]
    n167 = call "Sub_truncate_buffer.vi"("array"=w135, "samples"=w128) -> ("array"=w115:dbl[])  [unwired: 9 in]
    n168 = call "Sub_truncate_buffer.vi"("array"=w130, "samples"=w128) -> ("array"=w134:dbl[])  [unwired: 9 in]
    n169 = call "Sub_truncate_buffer.vi"("array"=w129, "samples"=w128) -> ("array"=w116:dbl[])  [unwired: 9 in]
    n170 = Subtract(x=w122, y=w124) -> (x-y=w123:dbl)
    n171 = Absolute Value(x=w123) -> (abs(x)=w121:dbl)
    n172 = Array Max & Min(array=w115) -> (max value=→"max value":dbl, min value=→"min value":dbl)  [unwired: 2 out]
    n173 = Multiply(x=w121, y=1000.0) -> (x*y=→"Cycle time (ms)":dbl)
  }
  n174 = call <vilib>:"DAQmx Clear Task.vi"("task in"=w82, "error in"=w81) -> ()  [unwired: 13 in, 1 out]
  n175 = call "Sub_time_constant_start_2022.vi"("time_frequency_calculations_start"=w67, "time_accelerometer_acquire_start"=w64, "Experimental Results IN"=w61, "time_subsample_start"=w66, "time_FEA_end"=w63, "time_frequency_calculations_end"=w68, "time_compare_start"=w69, "measured_pin_location_tt"=w24, "time_cycle_end"=w65, "time_cycle_start"=w70, "time_FEA_start"=w29) -> ("Experimental Results OUT"=w40:T6)  [unwired: 8 in]
  n176 = Unbundle By Name(w59) -> ("beam_length"=w58:dbl, "number_of_FEA_nodes"=w60:i32)
  n177 = Unbundle By Name(w40) -> ("time_average_cycle"=w2:dbl)
  n178 = Decrement(x=w60) -> (x-1=w57:i32)
  n179 = Format Date/Time String() -> (date/time string=w74:string)  [unwired: 3 in]
  n180 = Divide(x=w58, y=w57) -> (x/y=w56:dbl)
  n181 = Multiply(x=w28, y=w56) -> (x*y=w3:dbl[])
  n182 = Bundle By Name("Y"=w5, "dt"=w2) -> (w39:waveform(dbl))  [unwired: 1 in]
  n183 = Bundle By Name("Y"=w27, "dt"=w2) -> (w38:waveform(dbl))  [unwired: 1 in]
  n184 = Bundle By Name("Y"=w4, "dt"=w2) -> (w8:waveform(dbl))  [unwired: 1 in]
  n185 = Bundle By Name("Y"=w3, "dt"=w2) -> (w7:waveform(dbl))  [unwired: 1 in]
  n186 = Multiply(x=1000.0, y=w2) -> (x*y=→"average cycle time (ms)":dbl)
  n187 = Build Array(w39, w38) -> (→"1st Nat. Freq. (Hz) 4":waveform(dbl)[])
  n188 = Build Array(w8, w7) -> (→"1st Nat. Freq. (Hz) 5":waveform(dbl)[])
  n189 = Bundle By Name(cluster=w40, "measured_frequency"=w5, "date_time"=w74, "estimated_pin_node"=w28, "estimated_frequency"=w27, "estimated_pin_location"=w3, "measured_pin_location"=w4) -> (w43:T6)
  n190 = case shown="True" "Save Acceleration Data" {
    tunnel: [w441 w448] -> w42
    tunnel: w43 -> [w441 w447]
    tunnel: w41 -> [_ w446]
    tunnel: w26 -> [_ _]
    tunnel: w25 -> [_ _]
    frame False {
    }
    frame True {
      n191 = Unbundle By Name(w447) -> ("accelerometer_sample_rate"=w442:dbl)
      n192 = Reciprocal(x=w442) -> (1/x=w443:dbl)
      n193 = Array Size(array=w446) -> (size(s)=w444:i32)
      n194 = for {
        N: w444 -> [_]
        tunnel: w443 -> [w450]
        tunnel: [w449] -> w445 mode=indexing
        i -> [w451]
        n195 = Multiply(x=w450, y=w451) -> (x*y=w449:dbl)
      }
      n196 = Bundle By Name(cluster=w447, "time_acceleration_data"=w445, "acceleration_data"=w446) -> (w448:T6)
    }
  }
  n197 = flat-sequence {
    tunnel: w55 -> [w456]
    frame #0 {
      n198 = Unbundle By Name(w456) -> ("measured_pin_location_tt"=w467:dbl[], "measured_pin_location"=w455:dbl[], "time_cycle_end"=w466:dbl[], "estimated_pin_location"=w454:dbl[])
      n199 = Unbundle By Name(w456) -> ("measured_pin_location_tt"=w465:dbl[], "measured_pin_location"=w461:dbl[], "time_acceleration_data"=w452:dbl[], "acceleration_data"=w463:dbl[])
      n200 = Bundle("measured_pin_location_tt"=w467, "measured_pin_location"=w455) -> (w468:T13)  [unwired: 1 in]
      n201 = Bundle("time_acceleration_data"=w452, "acceleration_data"=w463) -> (w462:T14)  [unwired: 1 in]
      n202 = Multiply(x=w461, y=100.0 ("x")) -> (x*y=w458:dbl[])
      n203 = Bundle("time_cycle_end"=w466, "estimated_pin_location"=w454) -> (w453:T15)  [unwired: 1 in]
      n204 = Subtract(x=w458, y=6.8) -> (x-y=w457:dbl[])
      n205 = Bundle("measured_pin_location_tt"=w465, w457) -> (w464:cluster{"measured_pin_location_tt":dbl[], dbl[]})  [unwired: 1 in]
      n206 = Build Array(w464, w462) -> ()  [unwired: 1 out]
      n207 = Build Array(w468, w453) -> ()  [unwired: 1 out]
    }
  }
  n208 = flat-sequence {
    tunnel: w59 -> [w498]
    tunnel: w42 -> [w494]
    tunnel: "file name" -> [w489]
    tunnel: [w487] -> w55
    frame #0 {
      n209 = Unbundle(w494) -> ("time_average_cycle"=w499:dbl, "measured_frequency"=w500:dbl[], "date_time"=w501:string, "estimated_pin_node"=w502:i32[], "time_cycle_start"=w503:dbl[], "measured_pin_location"=w504:dbl[], "estimated_frequency"=w505:dbl[], "acceleration_data"=w506:dbl[], "accelerometer_sample_rate"=w507:dbl, "displacement_sample_rate"=w508:dbl, "time_compare_start"=w509:dbl[], "time_subsample_start"=w510:dbl[], "time_FEA_start"=w511:dbl[], "time_FEA_end"=w512:dbl[], "time_cycle_end"=w513:dbl[], "time_accelerometer_aquire_start"=w514:dbl[], "time_frequency_calculations_start"=w515:dbl[], "time_frequency_calculations_end"=w516:dbl[], "measured_pin_location_tt"=w497:dbl[], "time_ACC_data_collection_start"=w496:dbl, "time_acceleration_data"=w495:dbl[], "estimated_pin_location"=w488:dbl[], "scaling_factor_Hz_per_pin_to_frequency_resolution"=w486:dbl, "Std_Dev_equale_particles_divided_3"=w485:bool, "Auto_FFT_length"=w484:bool, "windowed_acc_data"=w483:dbl[][], "FFT"=w482:dbl[][])
      n210 = Unbundle(w498) -> ("beam_length"=w481:dbl, "youngs_modulus"=w480:dbl, "torsion_spring"=w479:dbl, "beam_height"=w478:dbl, "beam_width"=w477:dbl, "beam_density"=w476:dbl, "number_of_FEA_nodes"=w475:i32, "FFT_data_length"=w474:i32, "standard_deviation"=w473:dbl, "number_of_particles"=w472:i32, "min_FFT_power_value"=w471:dbl, "initial_pin_node"=w470:i32, "accelerometer_mass"=w469:dbl)  [unwired: 1 out]
      n211 = Number To Decimal String(number=w489) -> (decimal integer string=w490:string)  [unwired: 1 in]
      n212 = Current VI's Path() -> (path=w519:path)
      n213 = Strip Path(path=w519) -> (stripped path=w518:path)  [unwired: 1 out]
      n214 = Concatenate Strings("data\\data_" ("name or relative path"), w490, ".json" ("name or relative path")) -> (w491:string)
      n215 = Bundle("time_average_cycle"=w499, "measured_frequency"=w500, "date_time"=w501, "estimated_pin_node"=w502, "time_cycle_start"=w503, "measured_pin_location"=w504, "estimated_frequency"=w505, "acceleration_data"=w506, "accelerometer_sample_rate"=w507, "displacement_sample_rate"=w508, "time_compare_start"=w509, "time_subsample_start"=w510, "time_FEA_start"=w511, "time_FEA_end"=w512, "time_cycle_end"=w513, "time_accelerometer_aquire_start"=w514, "time_frequency_calculations_start"=w515, "time_frequency_calculations_end"=w516, "measured_pin_location_tt"=w497, "time_ACC_data_collection_start"=w496, "time_acceleration_data"=w495, "estimated_pin_location"=w488, "scaling_factor_Hz_per_pin_to_frequency_resolution"=w486, "Std_Dev_equale_particles_divided_3"=w485, "Auto_FFT_length"=w484, "windowed_acc_data"=w483, "FFT"=w482, "beam_length"=w481, "youngs_modulus"=w480, "torsion_spring"=w479, "beam_height"=w478, "beam_width"=w477, "beam_density"=w476, "number_of_FEA_nodes"=w475, "FFT_data_length"=w474, "standard_deviation"=w473, "number_of_particles"=w472, "min_FFT_power_value"=w471, "initial_pin_node"=w470, "accelerometer_mass"=w469) -> (w487:T16)  [unwired: 1 in]
      n216 = Build Path(base path=w518, name or relative path=w491) -> (appended path=w517:path)
      n217 = Flatten To JSON(anything=w487) -> (JSON string=w520:string)  [unwired: 2 in, 1 out]
      n218 = Write to Text File(file (use dialog)=w517, text=w520) -> (refnum out=w522:refnum<file>, error out=w521:errorcluster)  [unwired: 2 in, 1 out]
      n219 = Close File(refnum=w522, error in=w521) -> ()  [unwired: 2 out]
    }
  }
